vi "Safe Shooter Mode.vi"(10 "Ball Detected?":bool, 11 "Shooter Commands":T2={"Command"=enum."Prime Shooter", "Mode"=enum."Manual", "Shot Type"=enum."Batter Shot", "Override Trigger Sensor"=FALSE, "Override Angle?"=FALSE, "Hide From Death"=FALSE}) -> (1 "Trigger Power":dbl, 2 "Right Power":dbl, 3 "Left Power":dbl, 4 "RPM Ready?":bool, 5 "State":T1, 6 "Shooter Ready?":bool, 7 "Vision Ready?":bool)   [LabVIEW 2015]
uses:
  Common Code/Shooter Command Cluster.ctl
  Common Code/Shooter Commands.ctl
  Common Code/Shoot Modes Enum.ctl
  Common Code/Shot Type.ctl
  Common Code/Shooter State.ctl
  Common Code/Change Detect Int.vi
  Common Code/Change Detect Boolean.vi
  Robot Global Data.vi
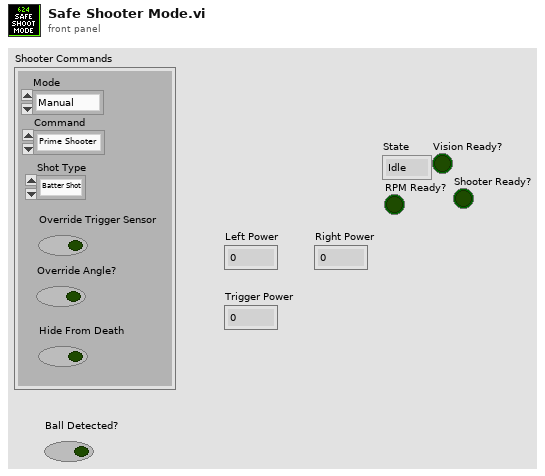
[diagram p1: front panel]
types:
  T1 = typedef "Shooter State.ctl" = enum16{"Idle", "Warmup", "Shooter Ready", "Shoot"}
  T2 = typedef "Shooter Command Cluster.ctl" = cluster{"Command":T3, "Mode":T4, "Shot Type":T5, "Override Trigger Sensor":bool, "Override Angle?":bool, "Hide From Death":bool}
  T3 = typedef "Shooter Commands.ctl" = enum16{"Idle", "Prime Shooter", "Shoot"}
  T4 = typedef "Shoot Modes Enum.ctl" = enum16{"Manual", "Safe", "Auto"}
  T5 = typedef "Shot Type.ctl" = enum16{"Batter Shot", "Corner Shot", "Cleat Shot", "Vision Shot", "Deep Middle Shot"}
  T6 = typedef "Drivetrain Status Cluster.ctl" = cluster{"Modes":T7, "Y (Throttle)":dbl, "X (Steer)":dbl, "Gyro In Range?":bool, "Distance Drive Finished?":bool, "Stop Eject Lockout":bool, "Dist Drive Status":T8, "Y Target":dbl, "Heading Target":dbl, "Vision Target Aligned?":bool, "Gear":dbl, "1st Gear Time":dbl, "2nd Gear Time":dbl, "1st Gear Shifts":dbl, "2nd Gear Shifts":dbl}
  T7 = typedef "Drivetrain Modes.ctl" = enum16{"Tank", "Climb", "Manual", "Goal Vision Targeting", "PID Distance Drive", "Hybrid", "Gyro Steer"}
  T8 = typedef "Dist Drive Status.ctl" = cluster{"Y In Range":bool, "X In Range":bool, "Gyro In Range":bool, "Y Dist":dbl, "X Dist":dbl, "Gyro":dbl}
  T9 = typedef "Dashboard Control Data.ctl" = cluster{"Shooter Presets":T10, "Encoder Control":T12, "Steer PID output":cluster{"output high":dbl, "output low":dbl}, " Steer PID gains":cluster{"proportional gain (Kc)":dbl, "integral time (Ti, min)":dbl, "derivative time (Td, min)":dbl}, "Drivetrain Settings":T13, "Vision Packet":T14, "Dashboard Drivetrain Command":T15, "Info/Command Cluster":T17, "Ball Vision Packet":T18, "Intake Presets":T20, "Intake Encoder Control":T22, "Climb Presets":T23, "Goal Output Range":cluster{"output high":dbl, "output low":dbl}, "Enabled Systems":T24, "Auton Presets":T25, "Pressure M":dbl, "Pressure B":dbl}
  T10 = typedef "Shooter Presets.ctl" = cluster{"Batter Shot":T11, "Deep Middle":T11, "Manual Shot":T11, "Left Ticks Per Rotation":dbl, "Right Ticks Per Rotation":dbl, "Low Bar Shot":T11, "Shooter RPM Tolerance":dbl, "Trigger Power":dbl, "Fire from Load Delay":i32, "Max Angle":dbl, "Min Angle":dbl, "Angle PID gains":cluster{"P":dbl, "I":dbl, "D":dbl}, "Angle Output":cluster{"output high":dbl, "output low":dbl}, "Shooter Angle Tolerance":dbl, "Vision Shoot x^2":dbl, "Vision Shoot x":dbl, "IR Let Go Timer":dbl, "Feed Forward Max Accel":dbl, "Feed Forward Kv":dbl, "Backwards Trigger":dbl, "Shot Finish Delay (ms)":dbl, "Angle Max Current":dbl, "Angle Current Trip Time":dbl, "Intake Angle":dbl, "Vision Shoot c":dbl, "Reset?":bool, "Button Release Delay":dbl, "Angle Pot x":dbl, "Angle Pot c":dbl, "Ignore Angle?":bool, "Max RPM":dbl, "Safty Frist Angle":dbl, "Intake Danger Height":dbl, "Angle Pot B":i32, "Angle Pot M":dbl, "FF Finish RPM":dbl, "RPM PID Right":cluster{"P":dbl, "I":dbl, "D":dbl, "FF":dbl}, "RPM PID Left":cluster{"P":dbl, "I":dbl, "D":dbl, "FF":dbl}, "Backwards RPM":dbl, "Vision RPM":dbl, "Run Wheels Backward Delay":u32, "Cleat Shot":T11}
  T11 = typedef "Shot Presets.ctl" = cluster{"L":dbl, "R":dbl, "A":dbl}
  T12 = typedef "Encoder Control.ctl" = cluster{"Right Tick Constant":dbl, "Left Tick Constant":dbl, "Reset?":bool, "Y Dist":cluster{"PID gains":cluster{"proportional gain (Kc)":dbl, "integral time (Ti, min)":dbl, "derivative time (Td, min)":dbl}}, "Y Stop Thresh":dbl, "Y Stop Speed":dbl}
  T13 = typedef "Drivetrain Settings.ctl" = cluster{"Gyro Tolerance":dbl, "Throttle Ramp (ms)":dbl, "Kv":dbl, "Ka":dbl, "Feed Forward P":dbl, "Feed Forward D":dbl, "Goal Vision PID gains":cluster{"proportional gain (Kc)":dbl, "integral time (Ti, min)":dbl, "derivative time (Td, min)":dbl}, "Goal Detection Window":dbl, "Creep Rate":dbl, "Vision Throttle Threshold":dbl, "Min Turn Output":dbl, "Left Batter Angle":dbl, "Right Batter Angle":dbl}
  T14 = typedef "Goal Vision Packet.ctl" = cluster{"Distance":dbl, "Center X":dbl, "Center Y":dbl, "Found Target?":bool, "Robot Center":dbl, "Angle":dbl}
  T15 = typedef "Dashboard Drivetrain Command.ctl" = cluster{"Drivetrain Vision":T16}
  T16 = typedef "Drivetrain Vision.ctl" = cluster{"Goal Window":dbl, "Ball Window":dbl}
  T17 = typedef "Ball Tracking Command Cluster.ctl" = cluster{"Distance to Ball":dbl, "Desired Angle":dbl, "Command":enum16{"Turn to Ball", "Turn to Angle", "Get Distance"}, "Pixels from Center":dbl}
  T18 = typedef "Ball Vision Packet.ctl" = cluster{"Ball Detected?":bool, "Distance to Ball":dbl, "Desired Angle":dbl, "Pixels from Center":dbl, "Tracking mode":T19}
  T19 = typedef "Tracking Mode.ctl" = enum16{"Turn to Ball", "Turn to Angle"}
  T20 = typedef "Intake Presets.ctl" = cluster{"Intake Speed":dbl, "Outake Speed":dbl, "Low Height":dbl, "Half Height":dbl, "Full Height":dbl, "Angle Speed":dbl, "Angle Tolerance":dbl, "Encoder Scale":dbl, "Load Height":dbl, "Output Range":T21, "Rotation Power Max/Min":dbl, "MaxCurrent":dbl, "Intake Trip Time":dbl, "Idle Height":dbl, "Max Height":dbl, "Reset Encoders?":bool, "PID gains":cluster{"proportional gain (Kc)":dbl, "integral time (Ti, min)":dbl, "derivative time (Td, min)":dbl}, "Intake Stop Delay":u32, "Settle Time":dbl, "Settle Wait Time":dbl}
  T21 = typedef "Drivetrain Output Range.ctl" = cluster{"output high":dbl, "output low":dbl}
  T22 = typedef "IntakeEcoderControl.ctl" = cluster{"Arm Tick Constant":dbl, "Reset?":bool, "Y Dist":cluster{"PID gains":cluster{"proportional gain (Kc)":dbl, "integral time (Ti, min)":dbl, "derivative time (Td, min)":dbl}}, "Y Stop Thresh":dbl, "Y Stop Speed":dbl}
  T23 = typedef "Climb Presets.ctl" = cluster{"Pull Power":dbl, "Extend Power":dbl}
  T24 = typedef "Enabled Systems.ctl" = cluster{"Shoot":bool, "Intake":bool, "DT":bool, "Gyro":bool, "100ms":bool, "US":bool}
  T25 = typedef "Autonomous Presets.ctl" = cluster{"Pitch Limit":dbl, "Roll Limit":dbl, "Start Position":dbl, "Cross Position":dbl}
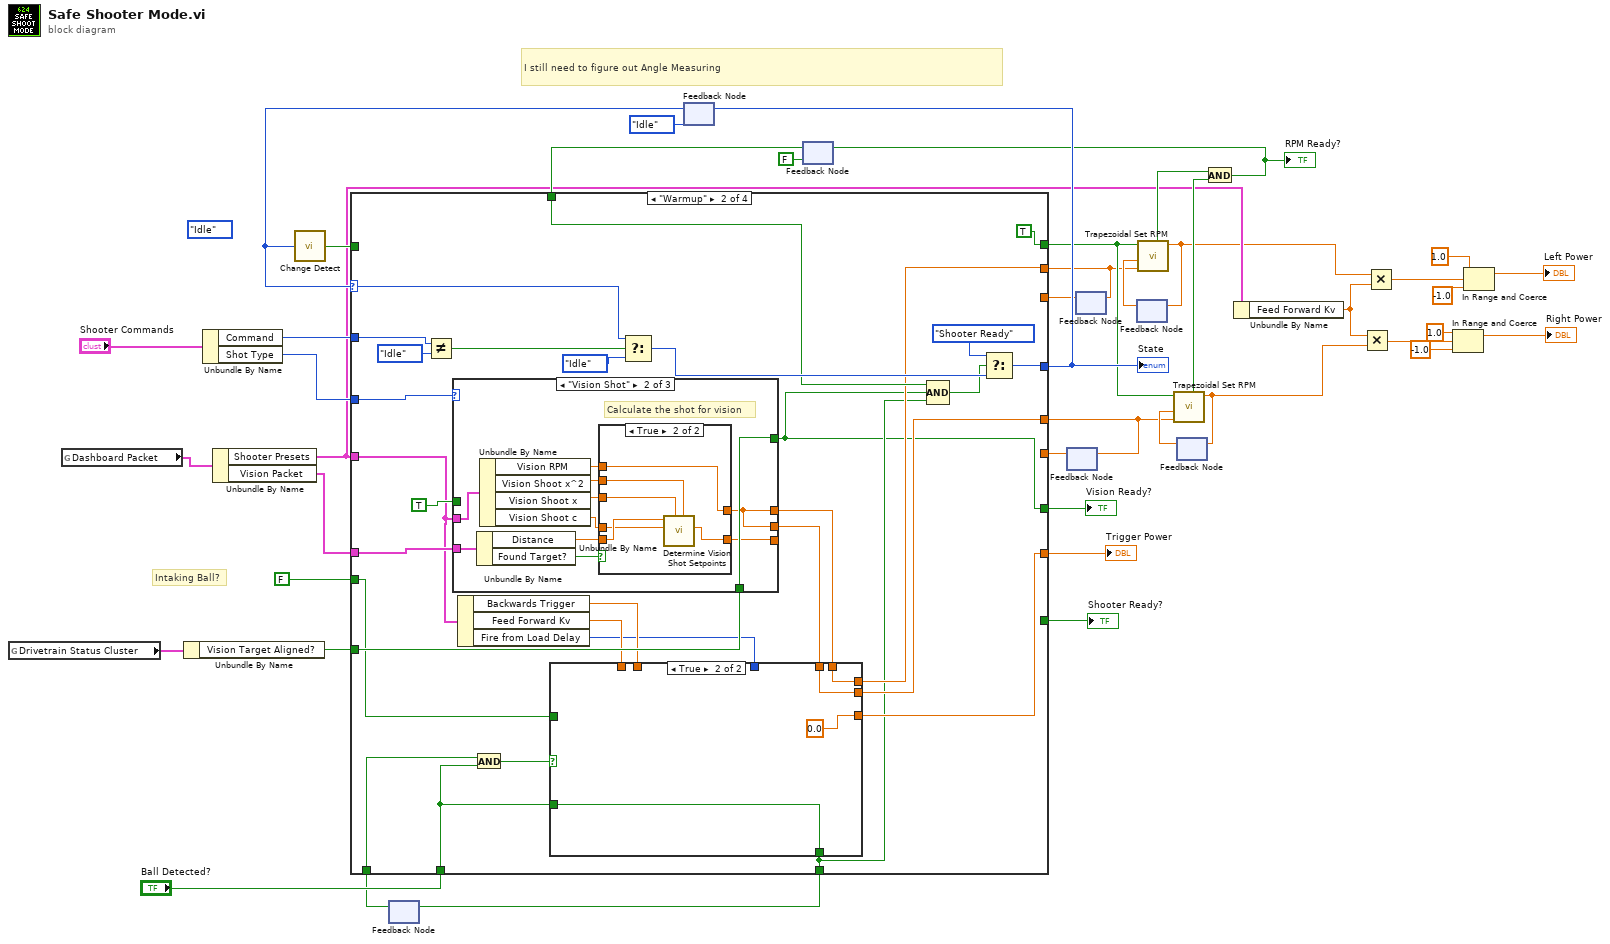
[diagram p0: block diagram]
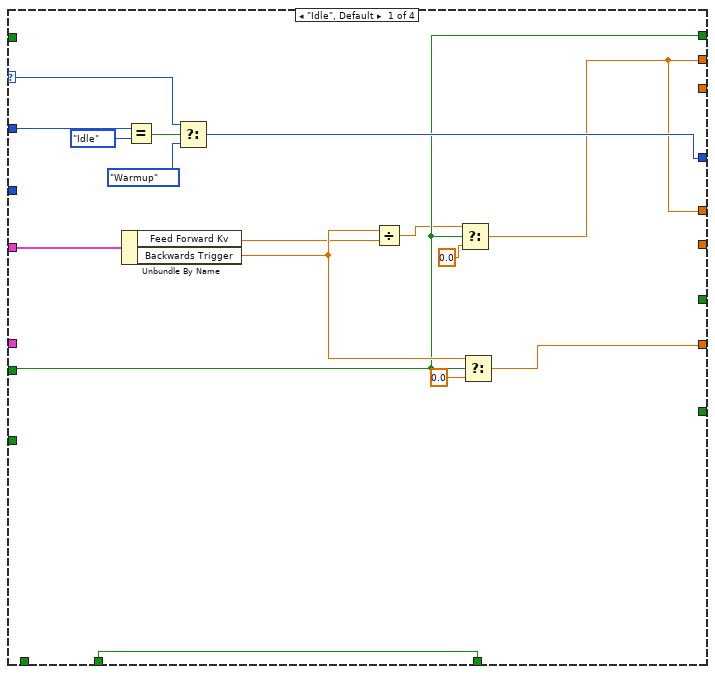
[diagram p2: hidden frame]
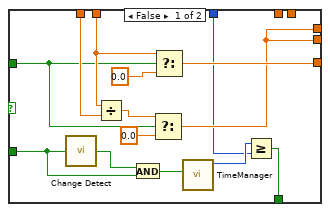
[diagram p3: hidden frame]
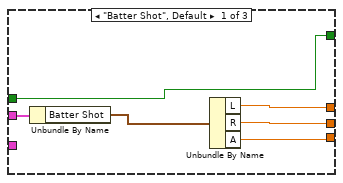
[diagram p4: hidden frame]
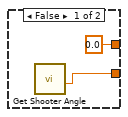
[diagram p5: hidden frame]
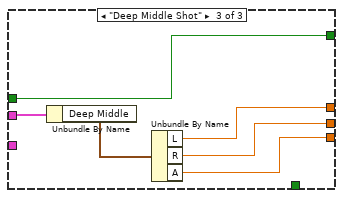
[diagram p6: hidden frame]
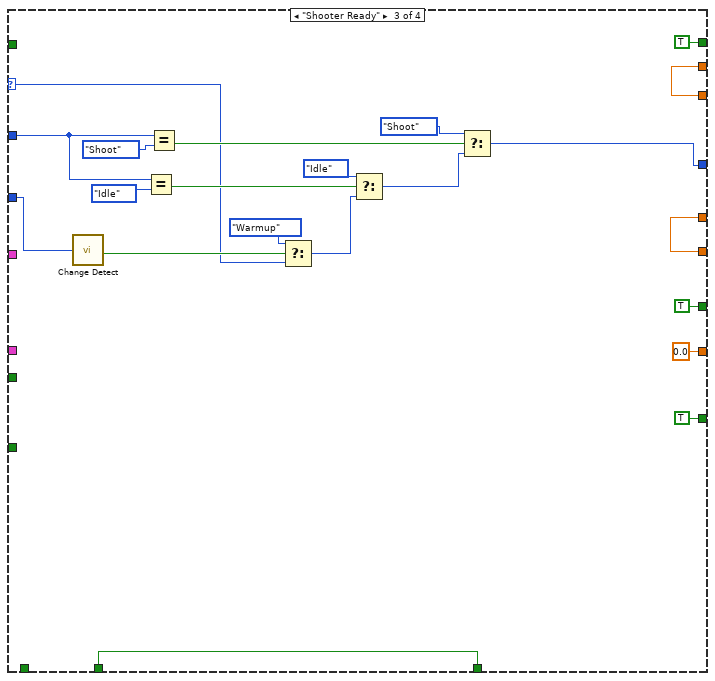
[diagram p7: hidden frame]
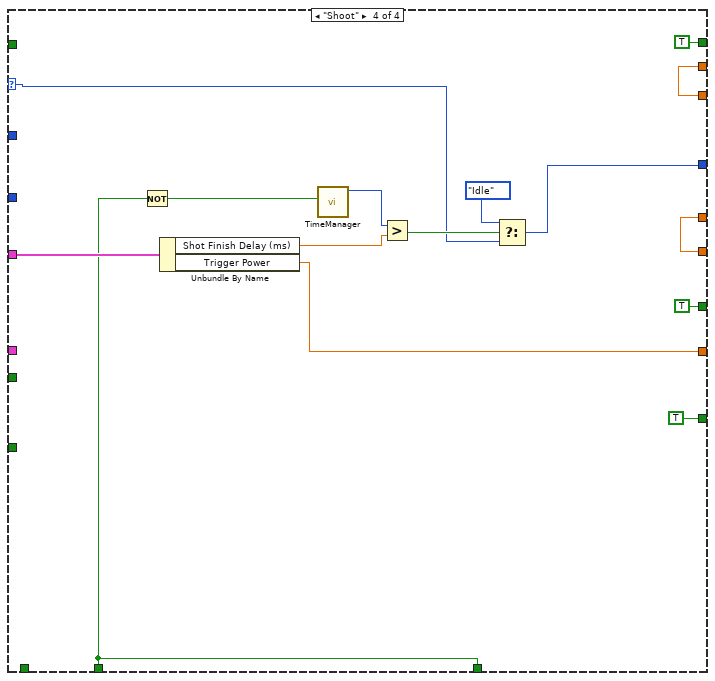
[diagram p8: hidden frame]
diagram:
  (unwired) Shooter_Commands."Idle" ("Command")
  # "I still need to figure out Angle Measuring"
  # "Intaking Ball?"
  n1 = global read "Robot Global Data.vi" "Drivetrain Status Cluster"() -> (w30:T6)
  n2 = global read "Robot Global Data.vi" "Dashboard Packet"() -> (w32:T9)
  n3 = Unbundle By Name(w30) -> ("Vision Target Aligned?"=w29:bool)
  n4 = Unbundle By Name("Shooter Commands") -> ("Command"=w36:T3, "Shot Type"=w33:T5)
  n5 = Unbundle By Name(w32) -> ("Shooter Presets"=w14:T10, "Vision Packet"=w31:T14)
  n6 = feedback #1() -> (w16:bool)  [unwired: 1 in]
  n7 = feedback #2(Shooter_State."Idle" ("Enum")) -> (w35:T1)
  n8 = call-poly "Change Detect.vi"("In"=w35) -> ("Changed?"=w34:bool)
  n9 = feedback #3(FALSE ("Shooter Ready?")) -> (w39:bool)
  n10 = feedback #4() -> (w22:dbl)  [unwired: 1 in]
  n11 = feedback #5() -> (w20:dbl)  [unwired: 1 in]
  n12 = case shown="\"Warmup\"" w35 {
    selector: w35 -> [w55 w84 w147 w164]
    tunnel: [w46 TRUE TRUE TRUE] -> w28
    tunnel: [w44 w69 w157 w172] -> w21
    tunnel: w39 -> [_ w75 _ _]
    tunnel: [w53 w80 w142 w162] -> w37
    tunnel: w36 -> [w58 w87 w152 _]
    tunnel: w34 -> [_ _ _ _]
    tunnel: w33 -> [_ w79 w149 _]
    tunnel: w14 -> [w52 w65 _ w170]
    tunnel: w31 -> [_ w78 _ _]
    tunnel: w29 -> [_ w76 _ _]
    tunnel: [w44 w68 w158 w171] -> w23
    tunnel: w22 -> [_ _ w158 w171]
    tunnel: w20 -> [_ _ w157 w172]
    tunnel: "Ball Detected?" -> [w43 w61 w140 w161]
    tunnel: [w50 w67 0.0 ("Trigger Power") w169] -> w19
    tunnel: FALSE -> [w46 w66 _ _]
    tunnel: w16 -> [_ w73 _ _]
    tunnel: [w43 w60 w140 w161] -> w15
    tunnel: [_ w59 TRUE ("Vision Target Aligned?") TRUE ("Vision Target Aligned?")] -> w2
    tunnel: [_ _ TRUE ("Vision Target Aligned?") TRUE ("Vision Target Aligned?")] -> w1
    frame "Idle", Default {
      n13 = Unbundle By Name(w52) -> ("Feed Forward Kv"=w48:dbl, "Backwards Trigger"=w49:dbl)
      n14 = Equal?(x=w58, y=Shooter_Commands."Idle") -> (x = y?=w56:bool)
      n15 = Select(t=w55, s=w56, f=Shooter_State."Warmup") -> (s? t:f=w53:T1)
      n16 = Divide(x=w49, y=w48) -> (x/y=w45:dbl)
      n17 = Select(t=w45, s=w46, f=0.0) -> (s? t:f=w44:dbl)
      n18 = Select(t=w49, s=w46, f=0.0) -> (s? t:f=w50:dbl)
    }
    frame "Warmup" {
      n19 = Not Equal?(x=w87, y=Shooter_Commands."Idle") -> (x != y?=w85:bool)
      n20 = case shown="\"Vision Shot\"" w79 {
        tunnel: w65 -> [w112 w122 w137]
        tunnel: [w110 w117 w135] -> w70
        tunnel: [w109 w117 w134] -> w71
        tunnel: w78 -> [_ w119 _]
        tunnel: [w108 w123 w133] -> w59
        tunnel: w76 -> [_ w123 _]
        tunnel: TRUE -> [w108 _ w133]
        tunnel: [w107 w118 w132] -> _
        frame "Batter Shot", Default {
          n21 = Unbundle By Name(w112) -> ("Batter Shot"=w111:T11)
          n22 = Unbundle By Name(w111) -> ("L"=w110:dbl, "R"=w109:dbl, "A"=w107:dbl)
        }
        frame "Vision Shot" {
          # "Calculate the shot for vision"
          n23 = Unbundle By Name(w119) -> ("Distance"=w121:dbl, "Found Target?"=w120:bool)
          n24 = Unbundle By Name(w122) -> ("Vision RPM"=w113:dbl, "Vision Shoot x^2"=w115:dbl, "Vision Shoot x"=w116:dbl, "Vision Shoot c"=w114:dbl)
          n25 = case shown="True" w120 {
            tunnel: w121 -> [_ w131]
            tunnel: [w124 w130] -> w118
            tunnel: [0.0 ("Power") w126] -> w117
            tunnel: w116 -> [_ w129]
            tunnel: w115 -> [_ w128]
            tunnel: w114 -> [_ w127]
            tunnel: w113 -> [_ w126]
            frame False {
              n26 = call "Get Shooter Angle.vi"() -> ("Current Angle"=w124:dbl)  [unwired: 10 in, 1 out]
            }
            frame True {
              n27 = call "Determine Vision Shot Setpoints.vi"("x^2"=w128, "x"=w129, "c"=w127, "Distance from Target"=w131) -> ("Angle"=w130:dbl)  [unwired: 7 in]
            }
          }
        }
        frame "Deep Middle Shot" {
          n28 = Unbundle By Name(w137) -> ("Deep Middle"=w136:T11)
          n29 = Unbundle By Name(w136) -> ("L"=w135:dbl, "R"=w134:dbl, "A"=w132:dbl)
        }
      }
      n30 = Unbundle By Name(w65) -> ("Backwards Trigger"=w64:dbl, "Feed Forward Kv"=w63:dbl, "Fire from Load Delay"=w62:i32)
      n31 = And(x=w73, y=w61) -> (x .and. y?=w72:bool)
      n32 = case shown="True" w72 {
        tunnel: w71 -> [_ w105]
        tunnel: w70 -> [_ w106]
        tunnel: [w95 w106] -> w69
        tunnel: [w95 w105] -> w68
        tunnel: [w101 0.0 ("Trigger Power")] -> w67
        tunnel: w66 -> [w97 _]
        tunnel: w64 -> [w100 _]
        tunnel: w63 -> [w99 _]
        tunnel: w62 -> [w90 _]
        tunnel: w61 -> [w91 w103]
        tunnel: [w89 w103] -> w60
        frame False {
          n33 = call-poly "Change Detect.vi"("In"=w91) -> ("Changed?"=w94:bool)
          n34 = Divide(x=w100, y=w99) -> (x/y=w98:dbl)
          n35 = And(x=w94, y=w91) -> (x .and. y?=w93:bool)
          n36 = Select(t=w98, s=w97, f=0.0) -> (s? t:f=w95:dbl)
          n37 = Select(t=w100, s=w97, f=0.0) -> (s? t:f=w101:dbl)
          n38 = call "TimeManager.vi"("Reset?"=w93) -> ("Time Since Reset"=w92:u32)  [unwired: 9 in, 1 out]
          n39 = Greater Or Equal?(x=w92, y=w90) -> (x >= y?=w89:bool)
        }
        frame True {
        }
      }
      n40 = Select(t=w84, s=w85, f=Shooter_State."Idle") -> (s? t:f=w83:T1)
      n41 = Compound Arithmetic op=AND(w75, w59, w60) -> (w74:bool)
      n42 = Select(t=Shooter_State."Shooter Ready", s=w74, f=w83) -> (s? t:f=w80:T1)
    }
    frame "Shooter Ready" {
      n43 = call-poly "Change Detect.vi"("In"=w149) -> ("Changed?"=w148:bool)
      n44 = Equal?(x=w152, y=Shooter_Commands."Idle") -> (x = y?=w151:bool)
      n45 = Equal?(x=w152, y=Shooter_Commands."Shoot") -> (x = y?=w155:bool)
      n46 = Select(t=Shooter_State."Warmup", s=w148, f=w147) -> (s? t:f=w145:T1)
      n47 = Select(t=Shooter_State."Idle", s=w151, f=w145) -> (s? t:f=w144:T1)
      n48 = Select(t=Shooter_State."Shoot", s=w155, f=w144) -> (s? t:f=w142:T1)
    }
    frame "Shoot" {
      n49 = Not(x=w161) -> (.not. x?=w168:bool)
      n50 = Unbundle By Name(w170) -> ("Shot Finish Delay (ms)"=w166:dbl, "Trigger Power"=w169:dbl)
      n51 = call "TimeManager.vi"("Reset?"=w168) -> ("Time Since Reset"=w167:u32)  [unwired: 9 in, 1 out]
      n52 = Greater?(x=w167, y=w166) -> (0:w165:bool)
      n53 = Select(t=Shooter_State."Idle", s=w165, f=w164) -> (s? t:f=w162:T1)
    }
  }
  "Trigger Power" <- w19
  "State" <- w37
  "Vision Ready?" <- w2
  "Shooter Ready?" <- w1
  n54 = feedback-in #1(w15) -> ()
  n55 = feedback-in #2(w37) -> ()
  n56 = feedback-in #4(w23) -> ()
  n57 = feedback-in #5(w21) -> ()
  n58 = feedback #6() -> (w40:dbl)  [unwired: 1 in]
  n59 = call "Trapezoidal Set RPM.vi"("Desired RPM"=w21, "Current RPM"=w40, "Spinning Wheels?"=w28) -> ("RPM"=w11:dbl, "Shooter Ready?"=w26:bool)  [unwired: 6 in, 1 out]
  n60 = feedback-in #6(w11) -> ()
  n61 = feedback #7() -> (w24:dbl)  [unwired: 1 in]
  n62 = call "Trapezoidal Set RPM.vi"("Desired RPM"=w23, "Current RPM"=w24, "Spinning Wheels?"=w28) -> ("RPM"=w12:dbl, "Shooter Ready?"=w27:bool)  [unwired: 6 in, 1 out]
  n63 = feedback-in #7(w12) -> ()
  n64 = And(x=w26, y=w27) -> (x .and. y?=w25:bool)
  "RPM Ready?" <- w25
  n65 = feedback-in #3(w25) -> ()
  n66 = Unbundle By Name(w14) -> ("Feed Forward Kv"=w13:dbl)
  n67 = Multiply(x=w13, y=w12) -> (x*y=w10:dbl)
  n68 = Multiply(x=w11, y=w13) -> (x*y=w4:dbl)
  n69 = In Range and Coerce(upper limit=1.0, x=w10, lower limit=-1.0) -> (coerced(x)=→"Right Power":dbl)  [unwired: 1 out]
  n70 = In Range and Coerce(upper limit=1.0, x=w4, lower limit=-1.0) -> (coerced(x)=→"Left Power":dbl)  [unwired: 1 out]
